vi "Array Functions.vi"() -> ()   [LabVIEW 2012]
panel:
  out "子数组":i32[](array[numeric])
  out "二维数组(Integer)":i32[][](array[numeric])
  out "一维数组(DBL)":dbl[](array[numeric])
  out "二维数组大小":i32[](array[numeric])
  out "一维数组大小":i32
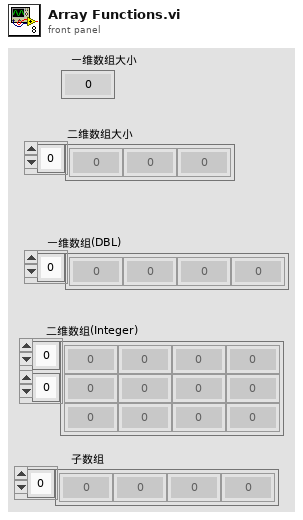
[diagram p1: front panel]
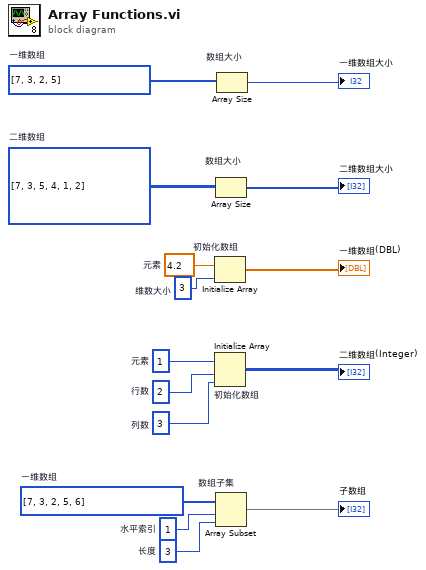
[diagram p0: block diagram]
diagram:
  w2 = 3  # 长度
  w3 = 1  # 水平索引
  w4 = i32[] [7, 3, 2, 5, 6]  # 一维数组
  w6 = 3  # 列数
  w7 = 2  # 行数
  w8 = 1  # 元素
  w10 = 3  # 维数大小
  w11 = 4.2  # 元素
  w13 = i32[][] [[7, 3, 5], [4, 1, 2]]  # 二维数组
  w15 = i32[] [7, 3, 2, 5]  # 一维数组
  n1 = Initialize Array "初始化数组"(w11, w10) -> (→"一维数组(DBL)":dbl[])
  n2 = Initialize Array "初始化数组"(w8, w7, w6) -> (→"二维数组(Integer)":i32[][])
  n3 = Array Size "数组大小"(array=w13) -> (size(s)=→"二维数组大小":i32[])
  n4 = Array Subset "数组子集"(array=w4, index=w3, length=w2) -> (→"子数组":i32[])
  n5 = Array Size "数组大小"(array=w15) -> (size(s)=→"一维数组大小":i32)
